vi "azimut.vi"() -> (0 "Numeric":u8)   [LabVIEW 2015, in "PolyVIEW.lvclass"]
uses:
  PolyVIEW.lvclass
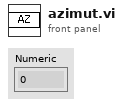
[diagram p1: front panel]
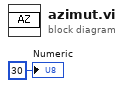
[diagram p0: block diagram]
diagram:
  "Numeric" <- u8 30
